vi "Load Config_Name Edits.vi"(8 "error in (no error)":errorcluster, 11 "Refnum in":T2) -> (0 "error out":errorcluster, 1 "Folder Name Edit":T1, 2 "File Name Edit":T1, 3 "Refnum out":T2)   [LabVIEW 2019, in "AutoMenuCreator.lvlib"]
uses:
  AutoMenuCreator.lvlib
  <vilib>/Utility/config.llb/Config Data RefNum.ctl
  Ctl/Ctl_Config_Name Edit.ctl
  <vilib>/Utility/config.llb/NI_LVConfig.lvlib
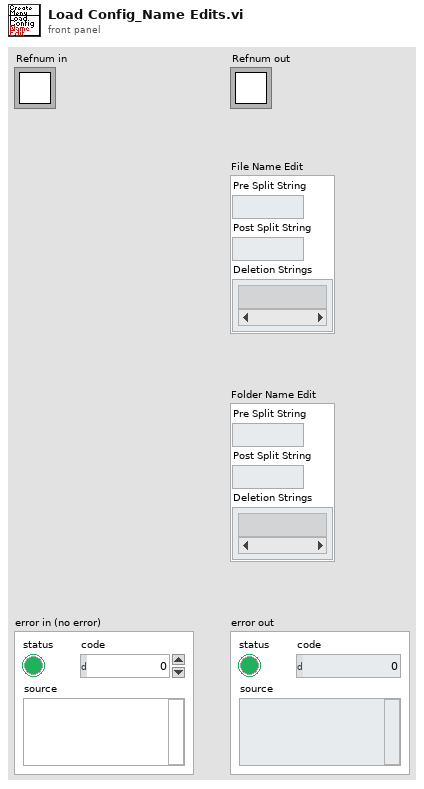
[diagram p1: front panel]
types:
  T1 = typedef "AutoMenuCreator.lvlib/Ctl_Config_Name Edit.ctl" = cluster{"Pre Split String":string, "Post Split String":string, "Deletion Strings":string[]}
  T2 = typedef "NI_LVConfig.lvlib/Config Data RefNum.ctl" = refnum<k1>
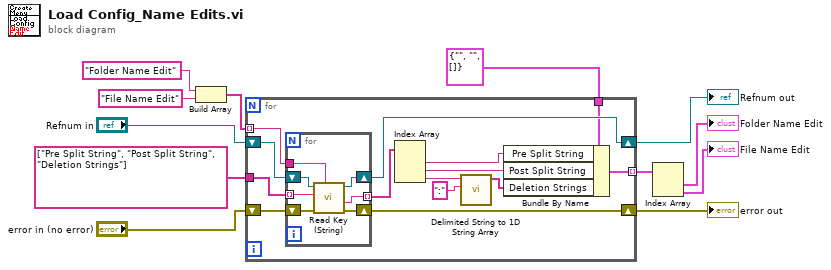
[diagram p0: block diagram]
diagram:
  n1 = Build Array("Folder Name Edit" ("section"), "File Name Edit" ("section")) -> (w3:string[])
  n2 = for {
    tunnel: [w19] -> w8 mode=indexing
    tunnel: w3 -> [w15] mode=indexing
    shift-right: [w23] -> w9
    shift-left: "error in (no error)" -> [w26]
    shift-right: [w24] -> w10
    shift-left: "Refnum in" -> [w25]
    tunnel: string[] ["Pre Split String", "Post Split String", "Deletion Strings"] ("key") -> [w14]
    tunnel: T1 {"Pre Split String"="", "Post Split String"="", "Deletion Strings"=[]} ("Folder Name Edit") -> [w13]
    n3 = for {
      tunnel: w15 -> [w31]
      shift-right: [w30] -> w24
      shift-left: w25 -> [w32]
      shift-right: [w29] -> w23
      shift-left: w26 -> [w33]
      tunnel: w14 -> [w28] mode=indexing
      tunnel: [w27] -> w22 mode=indexing
      n4 = call <vilib>:"Read Key (String).vi"("section"=w31, "error in (no error)"=w33, "key"=w28, "refnum"=w32) -> ("error out"=w29:errorcluster, "value"=w27:string, "refnum out"=w30:T2)  [unwired: 4 in, 1 out]
    }
    n5 = Index Array(array=w22) -> (element #1=w20:string, element #2=w21:string, element #3=w17:string)  [unwired: 3 in]
    n6 = call <vilib>:"Delimited String to 1D String Array.vi"("delimiter"=":", "delimited string"=w17) -> ("string array"=w16:string[])  [unwired: 9 in]
    n7 = Bundle By Name(cluster=w13, "Pre Split String"=w20, "Post Split String"=w21, "Deletion Strings"=w16) -> (w19:T1)
  }
  "error out" <- w9
  "Refnum out" <- w10
  n8 = Index Array(array=w8) -> (element #1=→"Folder Name Edit":T1, element #2=→"File Name Edit":T1)  [unwired: 2 in]
